vi "Code_to_run.vi"(0 "Extra command String":string, 1 "Open Front Panel":bool, 2 "Raw data option":enum16{"Save raw data", "Raw data not saved"}(ring), 3 "Current Row Comments":string, 4 "Camera Resolution":T1=1 items=["Low", "Med.", "High", "Max."], 5 "setup":T4, 7 "Remote control":bool, 9 "File":T2, 11 "Results Filename":path, 12 "Raw data file":path, 13 "Averaging time (min)":dbl=6.0 format="%.2f", 14 "Setup filename":string) -> (15 "Status":T3)   [LabVIEW 2015]
uses:
  Controls/Setup.ctl
  Multi_Run_Status.ctl
  Controls/Save_Data.ctl
  Camera Server/Camera enum/Camera resolution.ctl
  Controls/Post_Process.ctl
  Globals/Trav_pos_global.vi
  Globals/Meas_global.vi
  Globals/Constants_global.vi
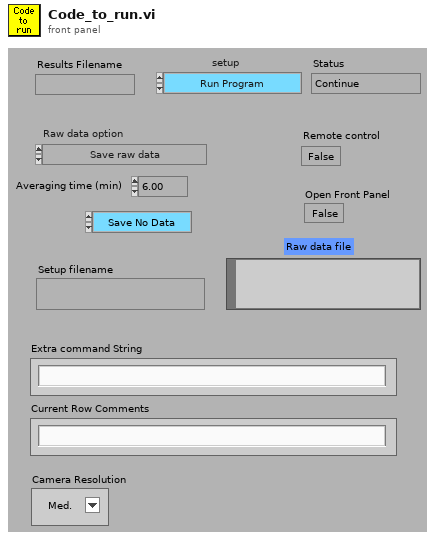
[diagram p1: front panel]
types:
  T1 = typedef "Camera resolution.ctl" = u8
  T2 = typedef "Save_Data.ctl" = enum16{"Save No Data", "Save Data"}
  T3 = typedef "Multi_Run_Status.ctl" = enum16{"Continue", "Jump to Next Point", "Jump to Next Row", "Jump To Fall Back", "Terminate Run"}
  T4 = typedef "Setup.ctl" = enum16{"Run Program", "Show Setup", "Save Current Setup", "Setup Front Panel"}
  T5 = typedef "Post_Process.ctl" = enum16{"Take New Data", "Post Process Raw Data File"}
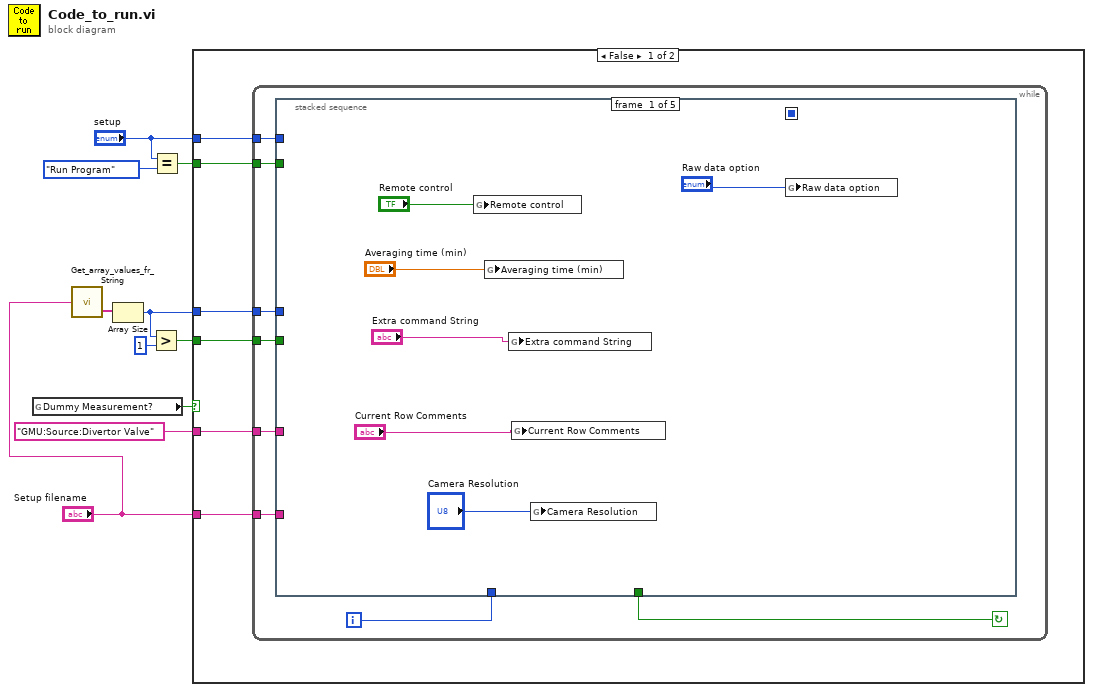
[diagram p0: block diagram]
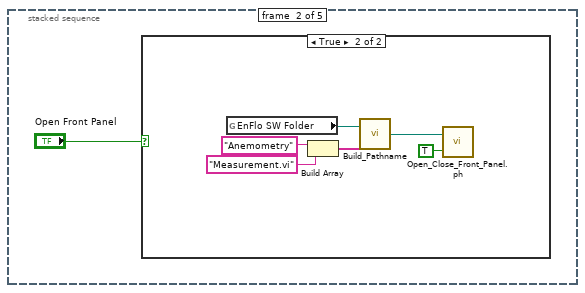
[diagram p2: hidden frame]
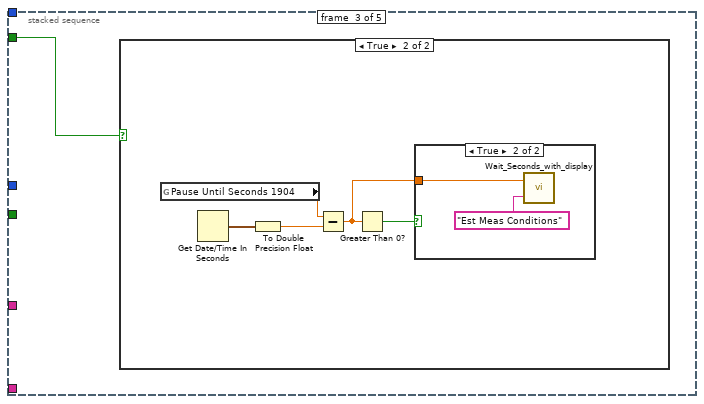
[diagram p4: hidden frame]
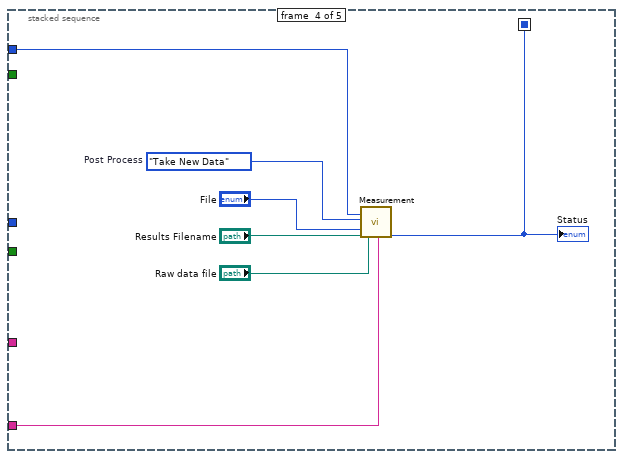
[diagram p7: hidden frame]
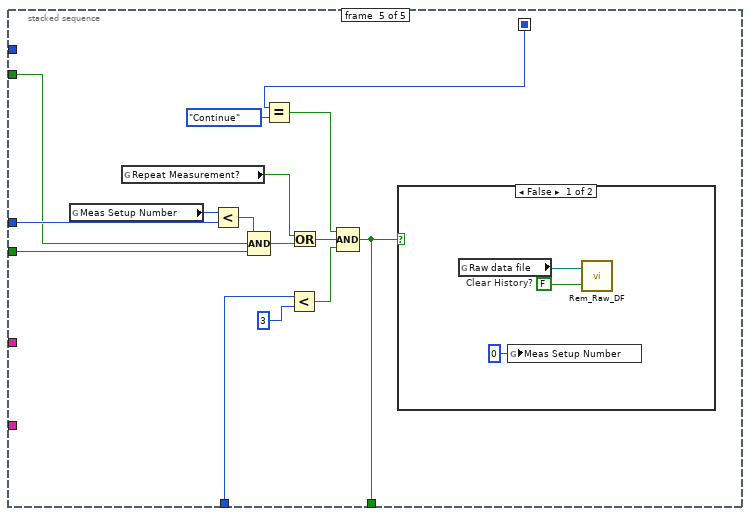
[diagram p8: hidden frame]
diagram:
  n1 = global read "Trav_pos_global.vi" "Dummy Measurement?"() -> (w10:bool)
  n2 = call "Get_array_values_fr_String.vi"("String Value"="Setup filename") -> ("String array"=w9:string[])  [unwired: 1 out]
  n3 = Array Size(array=w9) -> (size(s)=w7:i32)
  n4 = Greater?(x=w7, y=1) -> (0:w6:bool)
  n5 = Equal?(x="setup", y=Setup."Run Program" ("setup")) -> (x = y?=w3:bool)
  n6 = case shown="False" w10 {
    tunnel: w7 -> [w16 _]
    tunnel: w6 -> [w15 _]
    tunnel: "setup" -> [w14 _]
    tunnel: w3 -> [w13 _]
    tunnel: "GMU:Source:Divertor Valve" -> [w12 _]
    tunnel: "Setup filename" -> [w11 _]
    frame False {
      n7 = while {
        tunnel: w16 -> [w23]
        tunnel: w15 -> [w22]
        tunnel: w14 -> [w21]
        tunnel: w13 -> [w20]
        tunnel: w12 -> [w19]
        tunnel: w11 -> [w18]
        i -> [w17]
        stop <- w24 continue-if-true
        n8 = stacked-sequence {
          seq-local: [_ _ _ w48 _] -> [_ _ _ _ w66]
          tunnel: [_ _ _ _ w59] -> w24
          tunnel: w23 -> [_ _ _ _ w64]
          tunnel: w22 -> [_ _ _ _ w53]
          tunnel: w21 -> [_ _ _ w47 _]
          tunnel: w20 -> [_ _ w38 _ w54]
          tunnel: w19 -> [_ _ _ _ _]
          tunnel: w18 -> [_ _ _ w46 _]
          tunnel: w17 -> [_ _ _ _ w58]
          frame #0 {
            n9 = global write "Meas_global.vi" "Remote control"("Remote control") -> ()
            n10 = global write "Meas_global.vi" "Averaging time (min)"("Averaging time (min)") -> ()
            n11 = global write "Meas_global.vi" "Extra command String"("Extra command String") -> ()
            n12 = global write "Meas_global.vi" "Current Row Comments"("Current Row Comments") -> ()
            n13 = global write "Meas_global.vi" "Camera Resolution"("Camera Resolution") -> ()
            n14 = global write "Meas_global.vi" "Raw data option"("Raw data option") -> ()
          }
          frame #1 {
            n15 = case shown="True" "Open Front Panel" {
              frame False {
              }
              frame True {
                n16 = global read "Constants_global.vi" "EnFlo SW Folder"() -> (w34:path)
                n17 = Build Array("Anemometry", "Measurement.vi") -> (w35:string[])
                n18 = call "Build_Pathname.vi"("PathElements"=w35, "PathnameIn"=w34) -> ("AppendedPath"=w33:path)
                n19 = call "Open_Close_Front_Panel.ph.vi"("Front Panel Window:Open"=TRUE, "VI path"=w33) -> ()  [unwired: 2 out]
              }
            }
          }
          frame #2 {
            n20 = case shown="True" w38 {
              frame False {
              }
              frame True {
                n21 = global read "Trav_pos_global.vi" "Pause Until Seconds 1904"() -> (w43:dbl)
                n22 = Get Date/Time In Seconds() -> (seconds since 1Jan1904=w42:timestamp)
                n23 = To Double Precision Float(number=w42) -> (double precision float=w41:dbl)
                n24 = Subtract(x=w43, y=w41) -> (x-y=w39:dbl)
                n25 = Greater Than 0?(x=w39) -> (x > 0?=w40:bool)
                n26 = case shown="True" w40 {
                  tunnel: w39 -> [_ w44]
                  frame False {
                  }
                  frame True {
                    n27 = call "Wait_Seconds_with_display.vi"("Message"="Est Meas Conditions", "Seconds to wait"=w44) -> ()  [unwired: 2 out]
                  }
                }
              }
            }
          }
          frame #3 {
            w49 = Post_Process."Take New Data"  # Post Process
            n28 = call "Measurement.vi"("setup"=w47, "Post Process"=w49, "File"="File", "Results file"="Results Filename", "Raw data file"="Raw data file", "Setup filename"=w46) -> ("Status Out"=w48:T3)  [unwired: 1 in, 12 out]
            "Status" <- w48
          }
          frame #4 {
            n29 = global read "Trav_pos_global.vi" "Meas Setup Number"() -> (w65:i32)
            n30 = global read "Meas_global.vi" "Repeat Measurement?"() -> (w62:bool)
            n31 = Less?(x=w65, y=w64) -> (x < y?=w55:bool)
            n32 = Compound Arithmetic op=AND(w55, w54, w53) -> (w63:bool)
            n33 = Equal?(x=w66, y=Multi_Run_Status."Continue" ("Status Out")) -> (x = y?=w60:bool)
            n34 = Less?(x=w58, y=3) -> (x < y?=w56:bool)
            n35 = Or(x=w62, y=w63) -> (x .or. y?=w61:bool)
            n36 = Compound Arithmetic op=AND(w60, w61, w56) -> (w59:bool)
            n37 = case shown="False" w59 {
              frame False {
                w69 = FALSE  # Clear History?
                n38 = global read "Meas_global.vi" "Raw data file"() -> (w70:path)
                n39 = global write "Trav_pos_global.vi" "Meas Setup Number"(0 ("Meas Setup Number")) -> ()
                n40 = call "Rem_Raw_DF.vi"("Clear History?"=w69, "Filename to Remember"=w70) -> ()  [unwired: 1 out]
              }
              frame True {
              }
            }
          }
        }
      }
    }
    frame True {
    }
  }
